vi "Read Cell T2.vi"(8 "error in (no error)":errorcluster, 11 "cPAS Data in":refnum<class "cPAS Data.lvclass">) -> (0 "error out":errorcluster, 2 "T2":dbl, 3 "cPAS Data out":refnum<class "cPAS Data.lvclass">)   [LabVIEW 2015, in "cPAS Data.lvclass"]
uses:
  cPAS Data.lvclass
  cPAS Cell Data/cPAS Cell Data.lvclass
  Reusable/PAS/Data/Main/Read CellData.vi
  Reusable/PAS/Data/Main/Read Current Cell.vi
  Reusable/PAS/Data/Cell/PAS Cell Data.lvclass
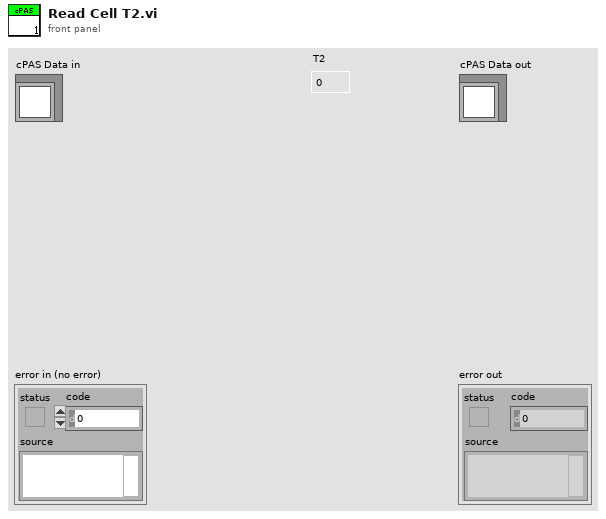
[diagram p1: front panel]
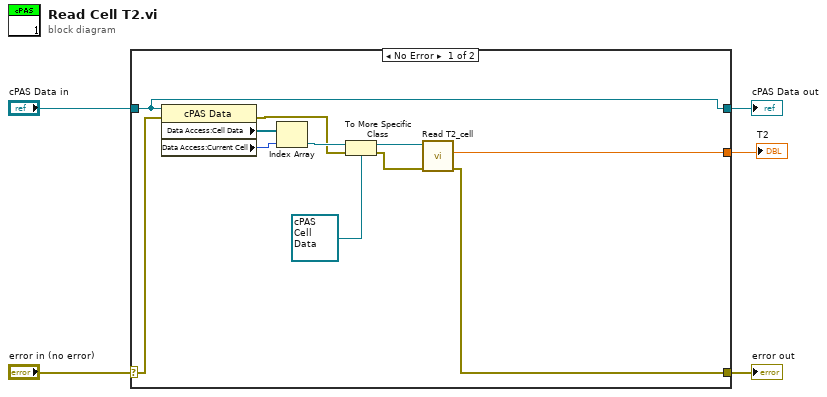
[diagram p0: block diagram]
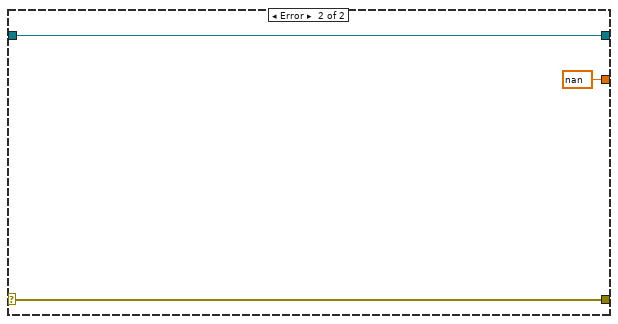
[diagram p2: hidden frame]
diagram:
  n1 = case shown="No Error" "error in (no error)" {
    selector: "error in (no error)" -> [w7 w19]
    tunnel: [w6 w19] -> w4
    tunnel: [w10 w18] -> w2
    tunnel: "cPAS Data in" -> [w10 w18]
    tunnel: [w8 nan ("T2")] -> w1
    frame No Error {
      n2 = property class="cPAS Data"(reference=w10, error in=w7) -> (error out=w13:errorcluster, "Data Access:Cell Data"=w16:refnum<class "PAS Cell Data.lvclass">[], "Data Access:Current Cell"=w15:i32)  [unwired: 1 out]
      n3 = Index Array(array=w16, index=w15) -> (element=w14:refnum<class "PAS Cell Data.lvclass">)
      n4 = To More Specific Class(target class=refnum<class "cPAS Cell Data.lvclass"> refnum ("cPAS Cell"), reference=w14, error in=w13) -> (specific class reference=w11:refnum<class "cPAS Cell Data.lvclass">, error out=w9:errorcluster)
      n5 = call "Read T2_cell.vi"("error in (no error)"=w9, "cPAS Cell in"=w11) -> ("error out"=w6:errorcluster, "T2"=w8:sgl)  [unwired: 7 in, 1 out]
    }
    frame Error {
    }
  }
  "error out" <- w4
  "cPAS Data out" <- w2
  "T2" <- w1
